vi "10_dosing.vi"() -> ()   [LabVIEW 2024]
uses:
  <vilib>/Utility/error.llb/DialogType.ctl
  4067e6f5-c9bb-441e-8d38-abed3cce061a.vi
  <vilib>/Utility/file.llb/Write Delimited Spreadsheet (DBL).vi
  <instrlib>/Tektronix DMM40x0 Series/Tektronix DMM40x0 Series.lvlib
panel:
  out "Array":dbl[](array[numeric])
  in  "stop":bool
  out "STABLE":bool
  in  "Serial Communication":T1={"Baud Rate"=9600, "Parity"=0, "Data Bits"=8, "Stop Bits"=10, "Flow Control"=0} {"Flow Control" items=["None", "XON/XOFF", "RTS/CTS", "XON/XOFF & RTS/CTS", "DTR/DSR", "XON/XOFF & DTR/DSR"]; "Stop Bits" items=["1.0"=10, "1.5"=15, "2.0"=20]; "Data Bits" items=["7"=7, "8"=8]; "Parity" items=["None", "Odd", "Even", "Mark", "Space"]; "Baud Rate" items=["300"=300, "600"=600, "1200"=1200, "2400"=2400, "4800"=4800, "9600"=9600, "19200"=19200]}
  out "Stability threshold":dbl format="%#_13g"
  out "Waveform Graph":dbl[](graph)
  # "Voltmeter Serial Configuration"
  # "DEFAULT SETTINGS:\n\nTimeout (10000 ms)\nTrigger Count (5000)\nSample Count (1)\n\n****DC VOLTAGE***"
  # "Voltmeter Stability"
  # "0 - Stability threshold not met\n1 - Stability threshold met\n\n\n\n*stability (+/-0.05 mV) of last 15 pts"
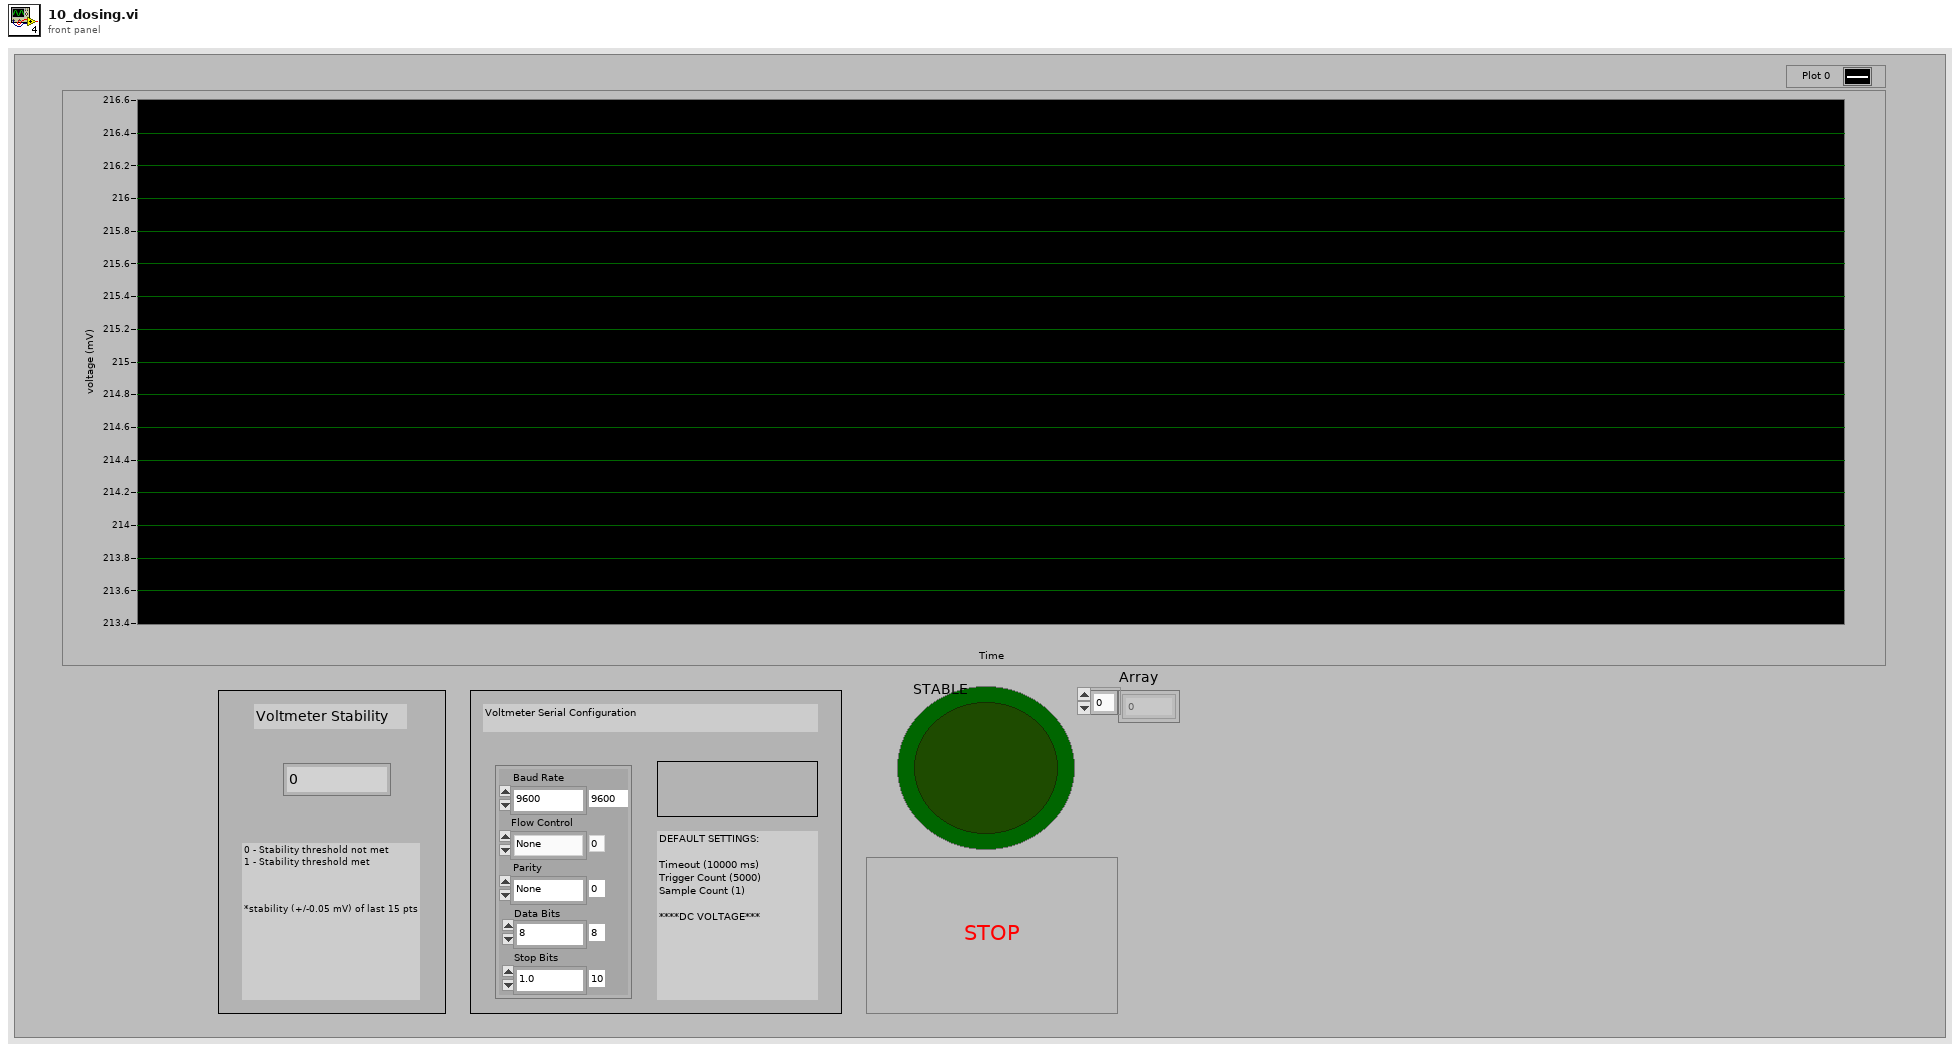
[diagram p1: front panel]
types:
  T1 = cluster{"Baud Rate":u32, "Parity":u16, "Data Bits":u16, "Stop Bits":u16, "Flow Control":u16}
  T2 = typedef "DialogType.ctl" = u16
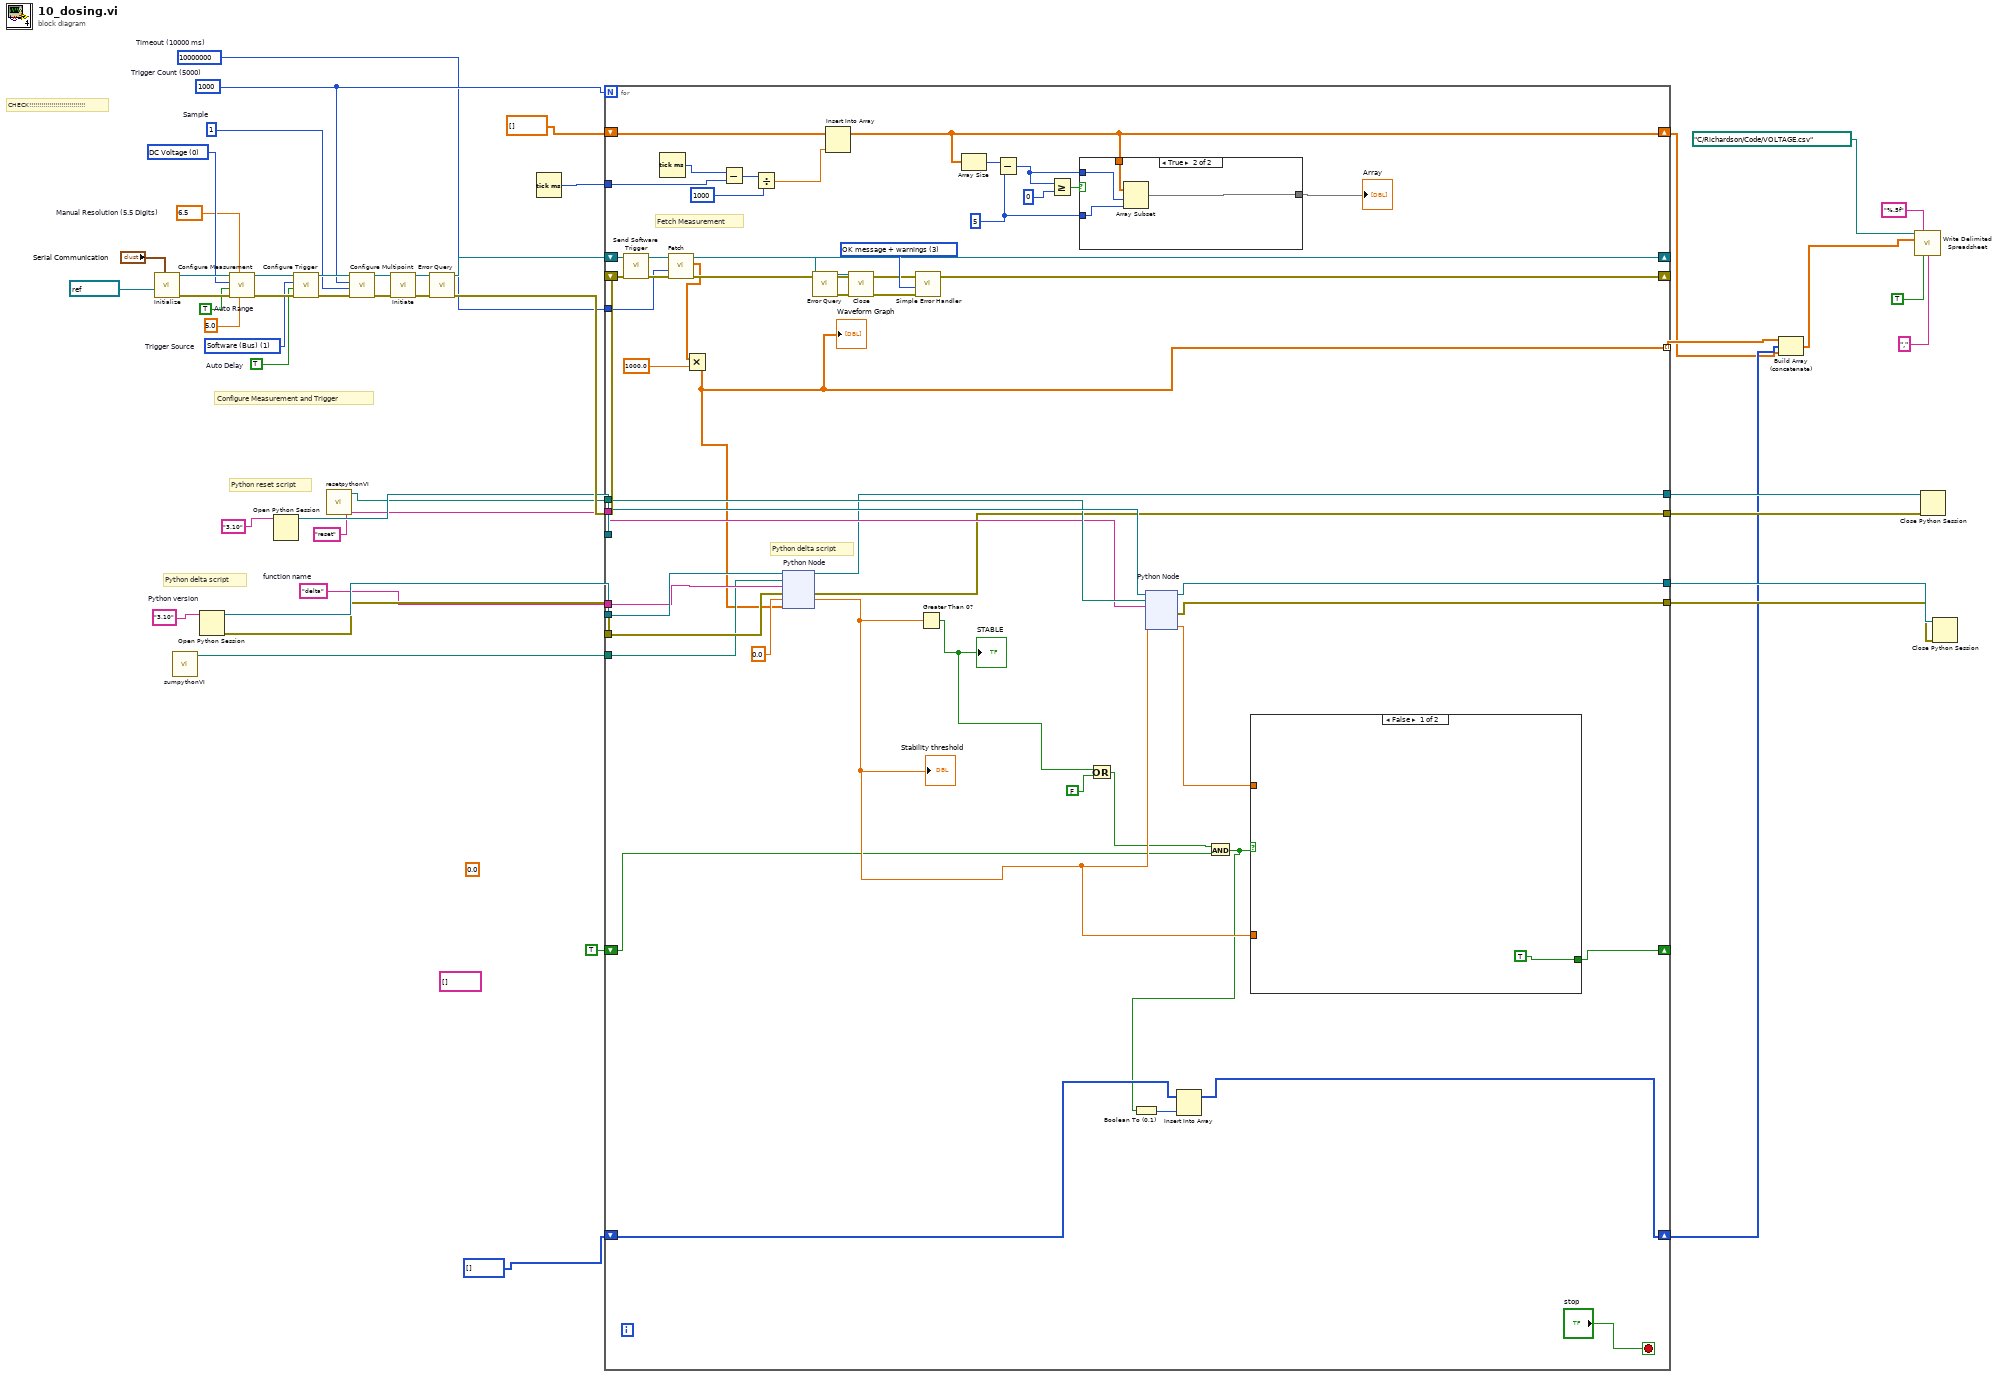
[diagram p0: block diagram]
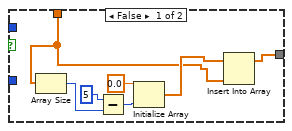
[diagram p2: hidden frame]
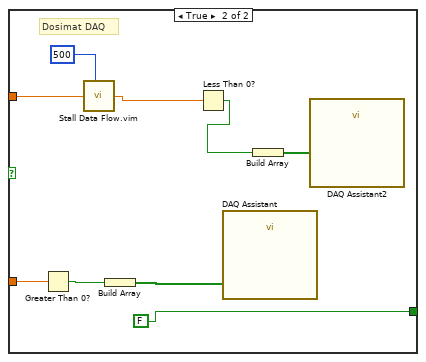
[diagram p3: hidden frame]
diagram:
  (unwired) 0.0
  (unwired) string[] []
  w14 = T2 3 items=["no dialog", "OK message", "continue or stop message", "OK message + warnings", "continue/stop + warnings"] ("type of dialog (OK msg:1)")
  w25 = "delta"  # function name
  w28 = "3.10"  # Python version
  w40 = u16 0 items=["DC Voltage", "AC Voltage", "2 - Wire Resistance", "4 - Wire Resistance", "DC Current", "AC Current", "Frequency", "Period", "Continuity", "Diode Checking", "Temperature", "Capacitance"] ("Function (0: DC Voltage)")
  w31 = u32 10000000  # Timeout (10000 ms)
  w32 = 1  # Sample
  w39 = 1000  # Trigger Count (5000)
  w33 = 6.5 items=["4.5"=4.5, "5.5"=5.5, "6.5"=6.5]  # Manual Resolution (5.5 Digits)
  w41 = TRUE  # Auto Delay
  w42 = u16 1 items=["Immediate", "Software (Bus)", "External"]  # Trigger Source
  w43 = TRUE  # Auto Range
  # "Python delta script"
  # "Python reset script"
  # "CHECK!!!!!!!!!!!!!!!!!!!!!!!!!!!!"
  # "Configure Measurement and Trigger"
  n1 = call <instrlib>:"Initialize.vi"("Serial Configuration"="Serial Communication", "VISA resource name"=refnum<visa-resource-name> "COM2" ("COM PORT (COM2)")) -> ("error out"=w52:errorcluster, "VISA resource name out"=w53:refnum<visa-resource-name>)  [unwired: 3 in, 5 out]
  n2 = call "sumpythonVI.vi"() -> ("appended path"=w24:path)  [unwired: 11 in]
  n3 = Open Python Session(python version=w28) -> (session out=w30:refnum<k35>, error out=w29:errorcluster)  [unwired: 2 in]
  n4 = call <instrlib>:"Configure Measurement.vi"("Manual Range (1.0)"=5.0, "Manual Resolution (5.5 Digits)"=w33, "error in (no error)"=w52, "Auto Range (T:Enable)"=w43, "Function (0: DC Voltage)"=w40, "VISA resource name"=w53) -> ("error out"=w50:errorcluster, "VISA resource name out"=w51:refnum<visa-resource-name>)  [unwired: 4 out]
  n5 = Open Python Session(python version="3.10" ("Python version")) -> (session out=w26:refnum<k35>)  [unwired: 2 in, 1 out]
  n6 = call <instrlib>:"Configure Trigger.vi"("error in (no error)"=w50, "Auto Delay (T: Enable)"=w41, "Trigger Source (0: Immediate)"=w42, "VISA resource name"=w51) -> ("error out"=w48:errorcluster, "VISA resource name out"=w49:refnum<visa-resource-name>)  [unwired: 1 in, 5 out]
  n7 = call "resetpythonVI.vi"() -> ("appended path"=w23:path)  [unwired: 11 in]
  n8 = call <instrlib>:"Configure Multipoint.vi"("error in (no error)"=w48, "Sample Count (1)"=w32, "Trigger Count (1)"=w39, "VISA resource name"=w49) -> ("error out"=w46:errorcluster, "VISA resource name out"=w47:refnum<visa-resource-name>)  [unwired: 6 out]
  n9 = call <instrlib>:"Initiate.vi"("error in (no error)"=w46, "VISA resource name"=w47) -> ("error out"=w38:errorcluster, "VISA resource name out"=w37:refnum<visa-resource-name>)  [unwired: 8 out]
  n10 = call <instrlib>:"Error Query.vi"("error in (no error)"=w38, "VISA resource name"=w37) -> ("error out"=w35:errorcluster, "VISA resource name out"=w36:refnum<visa-resource-name>)  [unwired: 8 out]
  n11 = Tick Count (ms)() -> (millisecond timer value=w3:u32)
  n12 = for {
    N: w39 -> [_]
    shift-right: [w99] -> _
    shift-left: w35 -> [w95]
    shift-right: [w100] -> w5
    shift-left: w36 -> [w96]
    tunnel: w31 -> [w94]
    tunnel: w30 -> [w89]
    tunnel: w29 -> [w88]
    tunnel: w26 -> [w87]
    tunnel: w25 -> [w86]
    tunnel: w24 -> [w85]
    tunnel: w23 -> [w84]
    tunnel: "reset" ("function name") -> [w83]
    tunnel: [w82] -> w21
    tunnel: [w81] -> w20
    tunnel: [w80] -> w19
    tunnel: [w79] -> w18
    shift-right: [w73] -> w7
    shift-left: i32[] [] -> [w74]
    tunnel: [w75] -> w8 mode=indexing
    shift-right: [w70] -> _
    shift-left: TRUE -> [w69]
    tunnel: w3 -> [w65]
    shift-right: [w55] -> w1
    shift-left: dbl[] [] -> [w61]
    stop <- "stop" stop-if-true
    w57 = 5 ("y")
    # "Python delta script"
    # "Fetch Measurement"
    n13 = call <instrlib>:"Send Software Trigger.vi"("error in (no error)"=w95, "VISA resource name"=w96) -> ("error out"=w97:errorcluster, "VISA resource name out"=w98:refnum<visa-resource-name>)  [unwired: 8 out]
    n14 = Tick Count (ms)() -> (millisecond timer value=w66:u32)
    n15 = call <instrlib>:"Fetch.vi"("error in (no error)"=w97, "Timeout (10000 ms)"=w94, "VISA resource name"=w98) -> ("error out"=w99:errorcluster, "Measurements"=w92:dbl[], "VISA resource name out"=w100:refnum<visa-resource-name>)  [unwired: 6 out]
    n16 = Multiply(x=w92, y=1000.0) -> (x*y=w75:dbl[])
    "Waveform Graph" <- w75
    n17 = Subtract(x=w66, y=w65) -> (x-y=w64:u32)
    n18 = Divide(x=w64, y=u32 1000) -> (x/y=w62:dbl)
    n19 = node "Python Node"(w89, w85, w86, w88, 0.0, w75) -> (w80:refnum<k35>, w79:errorcluster, w72:dbl)  [unwired: 1 in, 2 out]
    "Stability threshold" <- w72
    n20 = Insert Into Array(array=w61, new element=w62) -> (w55:dbl[])  [unwired: 1 in]
    n21 = Greater Than 0?(x=w72) -> (x > 0?=w76:bool)
    "STABLE" <- w76
    n22 = Array Size(array=w55) -> (size(s)=w60:i32)
    n23 = Subtract(x=w60, y=w57) -> (x-y=w56:i32)
    n24 = Greater Or Equal?(x=w56, y=0) -> (x >= y?=w59:bool)
    n25 = case shown="True" w59 {
      tunnel: w57 -> [_ w111]
      tunnel: w56 -> [_ w110]
      tunnel: w55 -> [w102 w109]
      tunnel: [w101 w108] -> w54
      frame False {
        n26 = Array Size(array=w102) -> (size(s)=w106:i32)
        n27 = Subtract(x=5, y=w106) -> (x-y=w107:i32)
        n28 = Initialize Array(0.0 ("element"), w107) -> (w103:dbl[])
        n29 = Insert Into Array(array=w103, new element=w102) -> (w101:dbl[])  [unwired: 1 in]
      }
      frame True {
        n30 = Array Subset(array=w109, index=w110, length=w111) -> (w108:dbl[])
      }
    }
    "Array" <- w54
    n31 = Or(x=w76, y=FALSE) -> (x .or. y?=w71:bool)
    n32 = node "Python Node"(w87, w84, w83, w72) -> (w82:refnum<k35>, w81:errorcluster, w90:dbl)  [unwired: 3 in, 2 out]
    n33 = And(x=w71, y=w69) -> (x .and. y?=w67:bool)
    n34 = Boolean To (0,1)(Boolean=w67) -> (0, 1=w68:i16)
    n35 = Insert Into Array(array=w74, new element=w68) -> (w73:i32[])  [unwired: 1 in]
    n36 = case shown="False" w67 {
      tunnel: w90 -> [_ w116]
      tunnel: w72 -> [_ w114]
      tunnel: [TRUE FALSE] -> w70
      frame False {
      }
      frame True {
        # "Dosimat DAQ"
        n37 = Greater Than 0?(x=w114) -> (x > 0?=w119:bool)
        n38 = call "Stall Data Flow.vim"("value in"=w116, "milliseconds to wait"=u32 500) -> ("value out"=w117:dbl)  [unwired: 1 out]
        n39 = Build Array(w119) -> (w118:bool[])
        n40 = Less Than 0?(x=w117) -> (x < 0?=w120:bool)
        n41 = call "DAQ Assistant"("data"=w118) -> ()  [unwired: 17 in, 2 out]
        n42 = Build Array(w120) -> (w121:bool[])
        n43 = call "DAQ Assistant2"("data"=w121) -> ()  [unwired: 17 in, 2 out]
      }
    }
  }
  n44 = call <instrlib>:"Error Query.vi"("VISA resource name"=w5) -> ("error out"=w15:errorcluster, "VISA resource name out"=w16:refnum<visa-resource-name>)  [unwired: 1 in, 8 out]
  n45 = call <instrlib>:"Close.vi"("error in (no error)"=w15, "VISA resource name"=w16) -> ("error out"=w17:errorcluster)  [unwired: 9 out]
  n46 = call <vilib>:"Simple Error Handler.vi"("type of dialog (OK msg:1)"=w14, "error in (no error)"=w17) -> ()  [unwired: 8 out]
  n47 = Build Array (concatenate)(w8, w7, w1) -> (w9:dbl[][])
  n48 = call-poly <vilib>:"Write Delimited Spreadsheet.vi"("file path (dialog if empty)"=path "C:/Richardson/Code/VOLTAGE.csv", "format (%.3f)"="%.5f", "2D data"=w9, "transpose? (no:F)"=TRUE, "delimiter (\\t)"="," ("delimiter (\\t)")) -> ()  [unwired: 9 in, 2 out]
  n49 = Close Python Session(session in=w19, error in=w18) -> ()  [unwired: 1 out]
  n50 = Close Python Session(session in=w21, error in=w20) -> ()  [unwired: 1 out]
